vi "Get(array).vi"(8 "error in (no error)":errorcluster, 10 "Path Array":string[](array[string]), 11 "JSON Value in":refnum<class "JSON Value.lvclass">) -> (0 "error out":errorcluster, 2 "JSON Value out":refnum<class "JSON Value.lvclass">, 3 "JSON Value out":refnum<class "JSON Value.lvclass">)   [LabVIEW 2016, in "JSON Value.lvclass"]
uses:
  JSON Value.lvclass
  Object/Get Value/Get Value (Value).vi
  Array/Index Array/Index Array (Value).vi
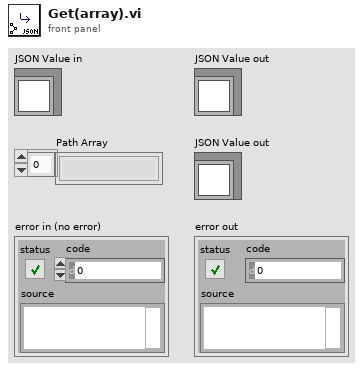
[diagram p1: front panel]
types:
  T1 = typedef "JSON Value.lvclass/JSON Types.ctl" = enum16{"String", "Numeric", "Boolean", "NULL", "Object", "Array"}
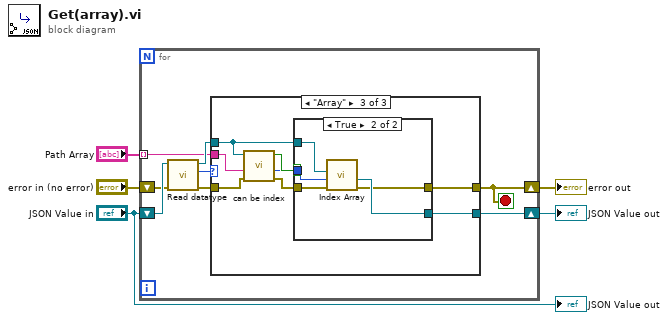
[diagram p0: block diagram]
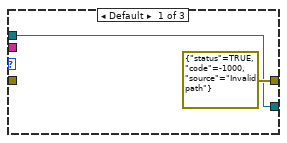
[diagram p2: hidden frame]
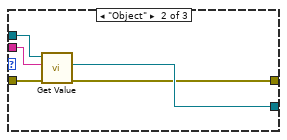
[diagram p3: hidden frame]
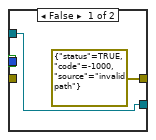
[diagram p4: hidden frame]
diagram:
  n1 = for {
    shift-right: [w9] -> w4
    shift-left: "JSON Value in" -> [w13]
    tunnel: "Path Array" -> [w10] mode=indexing
    shift-right: [w6] -> w1
    shift-left: "error in (no error)" -> [w7]
    stop <- w6 stop-if-true
    n2 = call "Read datatype.vi"("error in (no error)"=w7, "JSON Value in"=w13) -> ("error out"=w8:errorcluster, "datatype"=w12:T1, "JSON Value out"=w11:refnum<class "JSON Value.lvclass">)  [unwired: 7 in]
    n3 = case shown="\"Array\"" w12 {
      tunnel: w11 -> [w14 w20 w26]
      tunnel: w10 -> [_ w19 w25]
      tunnel: [w14 w18 w28] -> w9
      tunnel: w8 -> [_ w17 w24]
      tunnel: [errorcluster {"status"=TRUE, "code"=-1000, "source"="Invalid path"} ("error out") w16 w27] -> w6
      frame Default {
      }
      frame "Object" {
        n4 = call-poly "Get Value.vi"("error in (no error)"=w17, "key"=w19, "JSON Value in"=w20) -> ("error out"=w16:errorcluster, "JSON Value out"=w18:refnum<class "JSON Value.lvclass">)  [unwired: 7 in]
      }
      frame "Array" {
        n5 = call "can be index.vi"("error in (no error)"=w24, "string"=w25, "JSON Value in"=w26) -> ("error out"=w23:errorcluster, "index"=w21:i32, "valid index?"=w22:bool)  [unwired: 5 in, 1 out]
        n6 = case shown="True" w22 {
          tunnel: w26 -> [w30 w35]
          tunnel: [w30 w34] -> w28
          tunnel: [errorcluster {"status"=TRUE, "code"=-1000, "source"="invalid path"} ("error out") w33] -> w27
          tunnel: w23 -> [_ w32]
          tunnel: w21 -> [_ w31]
          frame False {
          }
          frame True {
            n7 = call-poly "Index Array.vi"("error in"=w32, "index"=w31, "JSON Value in"=w35) -> ("error out"=w33:errorcluster, "JSON Value out"=w34:refnum<class "JSON Value.lvclass">)  [unwired: 7 in]
          }
        }
      }
    }
  }
  "JSON Value out" <- w4
  "error out" <- w1
  "JSON Value out" <- "JSON Value in"
